vi "CustomSpectrum.vi"(0 "LightField Automation":refnum<class "LightField Automation.lvclass">, 1 "Photodiode handle out":refnum<visa-resource-name> caption="instrument handle out", 3 "Stop Spectrum Custom":refnum<vi>, 4 "Photodiode error out":errorcluster caption="error out" {"code" format="%.0x"}, 5 "LightField Automation error":errorcluster, 6 "CCD 1D Spectrum Main":refnum<vi>, 7 "Center Wavelength (nm)":refnum<vi>, 8 "Scan Spectrum Progess Bar":refnum<vi>, 10 "Excitation Power (uW)":refnum<vi>, 12 "Scan Spectrum Cust Exp Params 2":T1) -> (11 "WLs":dbl[](array[numeric]), 13 "PL":dbl[](array[numeric]), 14 "LFA Out":refnum<class "LightField Automation.lvclass">, 15 "PD Out":refnum<visa-resource-name>, 17 "movemonotime":u32, 18 "PD Error Our":errorcluster, 19 "LFA Error Out":errorcluster)   [LabVIEW 2019]
uses:
  C:/Users/manip/Documents/Controle_Manip_2020/Thorlabs.MotionControl.KCube.SolenoidCLI.dll
  Thorlabs.MotionControl.KCube.SolenoidCLI.dll
  Light Field/lightfield-automation-labview/LightField Automation.lvclass
  <vilib>/Analysis/baseanly.llb/Mean (DBL).vi
  <vilib>/Analysis/NI_AALBase.lvlib
panel:
  in  "Scan Spectrum Progess Bar":u8(slide) scale=0.0..100.0
  in  "Stop Spectrum Custom 2":bool
  in  "Stop Spectrum Custom":bool
  out "Array 2":i32[](array[numeric])
  out "Array":dbl[](array[numeric])
  out "Acq Time (ms)":dbl
  out "NumPoints":dbl
  out "KCube Shutter On?":bool
  out "Spectrum Custom Mode":u16
  out "Spectrum End Wavelength (nm)":dbl
  out "Spectrum Step Wavelength (nm)":dbl
  out "Spectrum Start Wavelength (nm)":dbl
  in  "Scan Spectrum Cust Exp Params":T2
  in  "Center Wavelength (nm)":dbl=490.12 caption="Center WL :"
  out "Excitation Power (uW)":dbl=0.2 caption="P    =" format="%#_3p"
  out "CCD 1D Spectrum Main":cluster{dbl[], dbl[]}(graph)
  out "Shutter Ctrls":u16(ring)
  out "KCube Shutter Device Reference":refnum<k24>
types:
  T1 = cluster{"Acq Time (ms)":dbl, "Spectrum Start Wavelength (nm)":dbl, "Spectrum Step Wavelength (nm)":dbl, "Spectrum End Wavelength (nm)":dbl, "Spectrum Custom Mode":u16, "KCube Shutter On?":bool}
  T2 = cluster{"Spectrum Start Wavelength (nm)":dbl, "Spectrum Step Wavelength (nm)":dbl, "Spectrum End Wavelength (nm)":dbl, "Spectrum Custom Mode":u16, "KCube Shutter On?":bool}
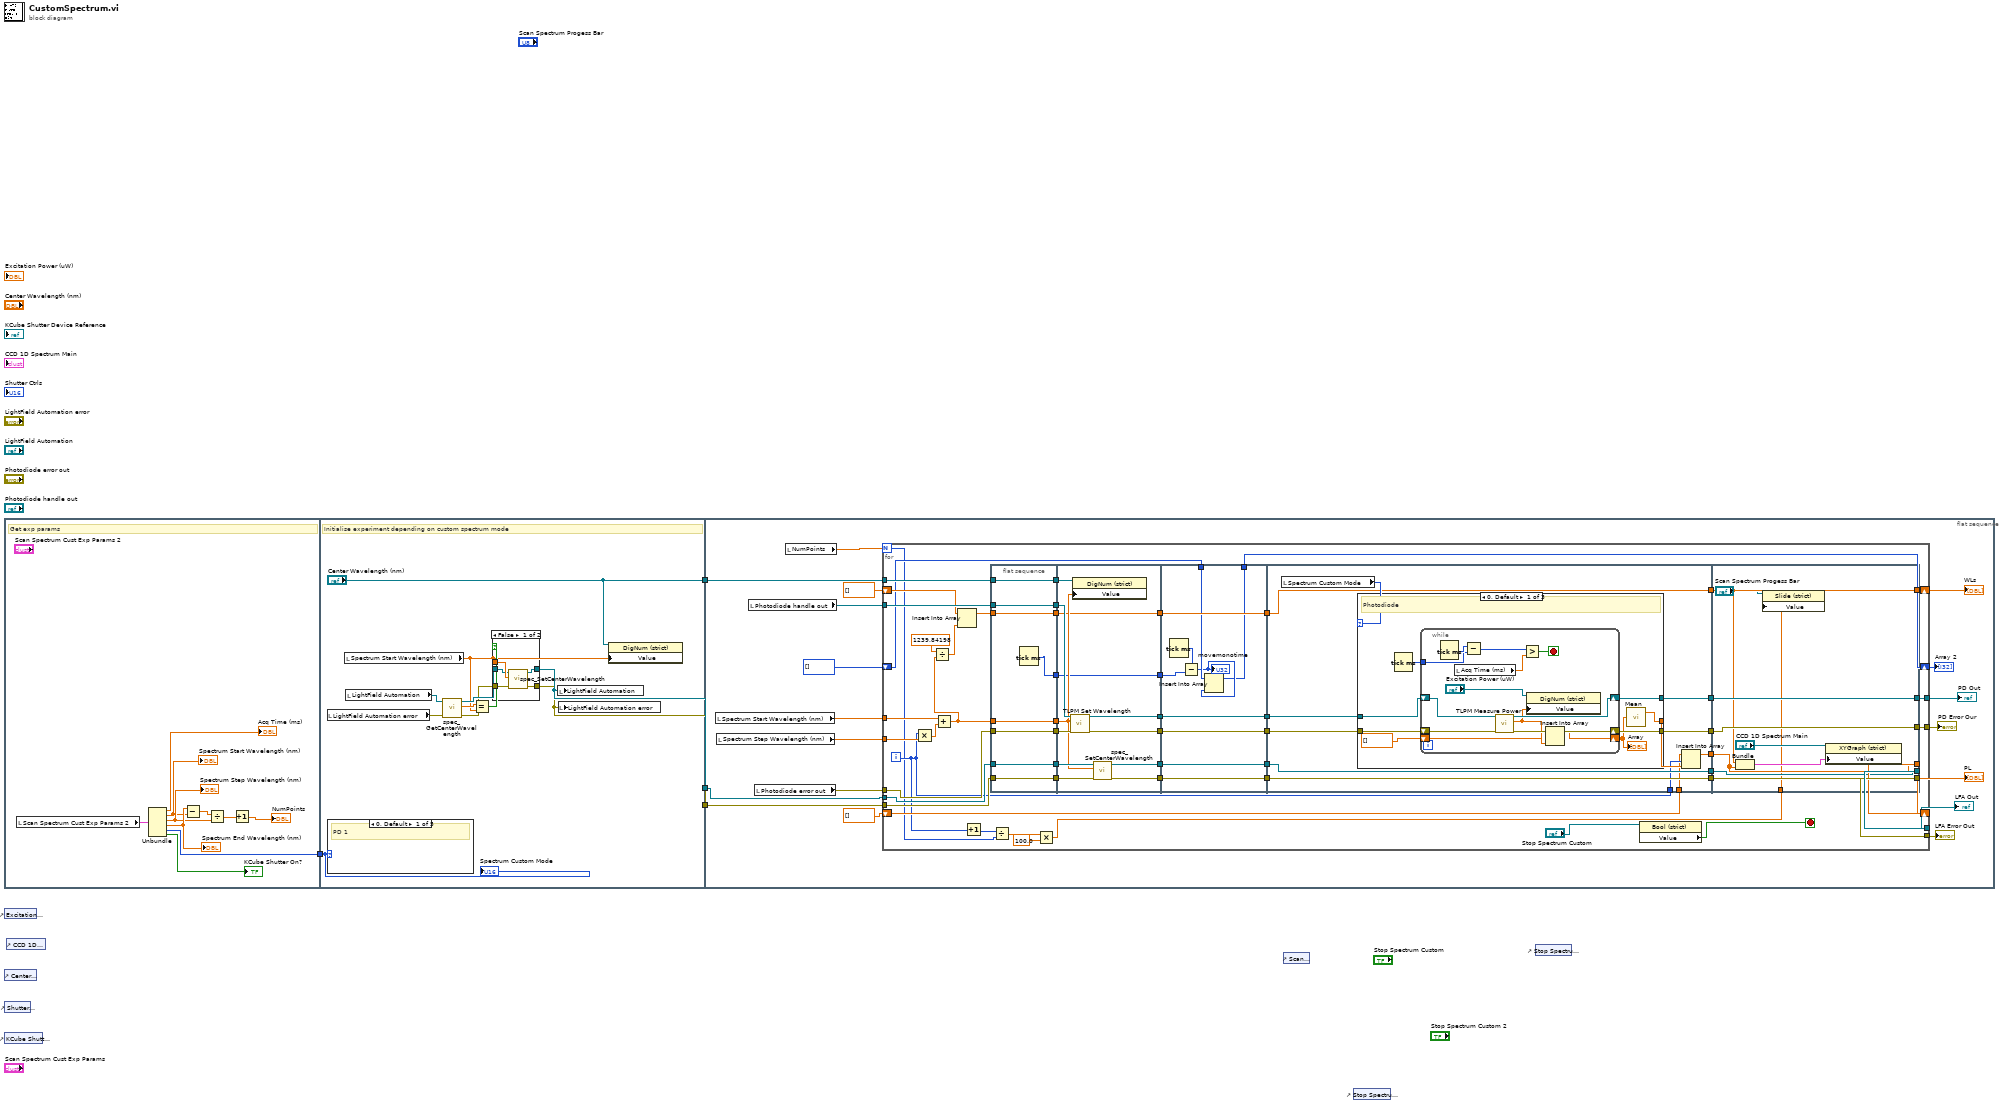
[diagram p0: block diagram]
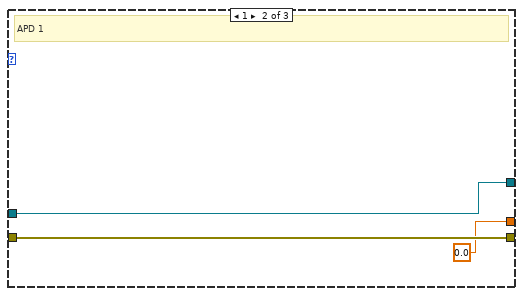
[diagram p7: hidden frame]
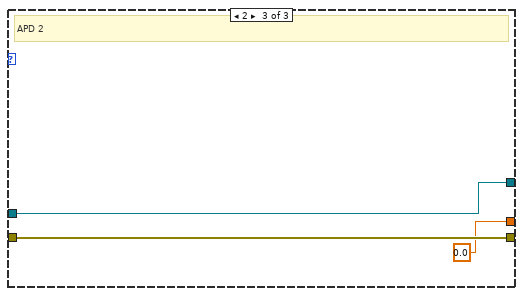
[diagram p8: hidden frame]
diagram:
  n1 = flat-sequence {
    tunnel: [w9] -> w4
    tunnel: w4 -> [w25]
    tunnel: [w17] -> w3
    tunnel: [w16] -> w2
    tunnel: ["Center Wavelength (nm)"] -> w1
    tunnel: w3 -> [w44]
    tunnel: w2 -> [w42]
    tunnel: w1 -> [w39]
    frame #0 {
      # "Get exp params"
      n2 = local read "Scan Spectrum Cust Exp Params 2"() -> (w14:T1)
      n3 = Unbundle(w14) -> ("Acq Time (ms)"=→"Acq Time (ms)":dbl, "Spectrum Start Wavelength (nm)"=w6:dbl, "Spectrum Step Wavelength (nm)"=w7:dbl, "Spectrum End Wavelength (nm)"=w8:dbl, "Spectrum Custom Mode"=w9:u16, "KCube Shutter On?"=→"KCube Shutter On?":bool)
      "Spectrum Start Wavelength (nm)" <- w6
      "Spectrum Step Wavelength (nm)" <- w7
      "Spectrum End Wavelength (nm)" <- w8
      n4 = Subtract(x=w8, y=w6) -> (x-y=w13:dbl)
      n5 = Divide(x=w13, y=w7) -> (x/y=w12:dbl)
      n6 = Increment(x=w12) -> (x+1=→"NumPoints":dbl)
    }
    frame #1 {
      # "Initialise experiment depending on custom spectrum mode"
      n7 = local read "LightField Automation error"() -> (w23:errorcluster)
      n8 = case shown="0, Default" w25 {
        frame 0, Default {
          # "PD 1"
        }
        frame 1 {
          # "APD 1"
        }
        frame 2 {
          # "APD 2"
        }
        frame 3 {
          # "APD 1+2"
        }
        frame 4 {
          # "PD 2"
        }
      }
      n9 = local read "Spectrum Start Wavelength (nm)"() -> (w18:dbl)
      n10 = local read "LightField Automation"() -> (w24:refnum<class "LightField Automation.lvclass">)
      n11 = call "spec_GetCenterWavelength.vi"("error in (no error)"=w23, "LightField Automation in"=w24) -> ("error out"=w19:errorcluster, "Center Wavelength"=w22:dbl, "LightField Automation out"=w20:refnum<class "LightField Automation.lvclass">)  [unwired: 7 in]
      n12 = Equal?(x=w22, y=w18) -> (x = y?=w21:bool)
      n13 = case shown="False" w21 {
        tunnel: w20 -> [w28 w32]
        tunnel: w19 -> [w29 w31]
        tunnel: [w27 w32] -> w17
        tunnel: [w26 w31] -> w16
        tunnel: w18 -> [w30 _]
        frame False {
          n14 = call "spec_SetCenterWavelength.vi"("error in (no error)"=w29, "Center Wavelength"=w30, "LightField Automation in"=w28) -> ("error out"=w26:errorcluster, "LightField Automation out"=w27:refnum<class "LightField Automation.lvclass">)  [unwired: 7 in]
        }
        frame True {
        }
      }
      n15 = local write "LightField Automation"(w17) -> ()
      n16 = local write "LightField Automation error"(w16) -> ()
      n17 = property class="DigNum (strict)"(reference="Center Wavelength (nm)", "Value"=w18) -> ()  [unwired: 1 in, 2 out]
      "Spectrum Custom Mode" <- w25
    }
    frame #2 {
      n18 = local read "Spectrum Start Wavelength (nm)"() -> (w49:dbl)
      n19 = local read "Spectrum Step Wavelength (nm)"() -> (w50:dbl)
      n20 = local read "Photodiode handle out"() -> (w45:refnum<visa-resource-name>)
      n21 = local read "Photodiode error out"() -> (w46:errorcluster)
      n22 = local read "NumPoints"() -> (w40:dbl)
      n23 = for {
        N: w40 -> [w57]
        tunnel: w50 -> [w104]
        tunnel: w49 -> [w103]
        tunnel: [w94] -> w48
        tunnel: [w93] -> w47
        tunnel: w46 -> [w92]
        tunnel: w45 -> [w91]
        tunnel: w44 -> [w90]
        tunnel: [w89] -> w43
        tunnel: w42 -> [w88]
        tunnel: [w87] -> w41
        tunnel: w39 -> [w86]
        shift-right: [w73] -> w36
        shift-left: dbl[] [] -> [w77]
        shift-right: [w74] -> w35
        shift-left: dbl[] [] -> [w75]
        shift-right: [w62] -> w33
        shift-left: i32[] [] -> [w63]
        i -> [w59]
        stop <- w60 stop-if-true
        n24 = Multiply(x=w59, y=w104) -> (x*y=w105:dbl)
        n25 = Add(x=w103, y=w105) -> (x+y=w52:dbl)
        n26 = Divide(x=1239.84198, y=w52) -> (x/y=w51:dbl)
        n27 = Insert Into Array(array=w77, new element=w51) -> (w76:dbl[])  [unwired: 1 in]
        n28 = Increment(x=w59) -> (x+1=w58:i32)
        n29 = flat-sequence {
          tunnel: w76 -> [w107]
          tunnel: w86 -> [w108]
          tunnel: w91 -> [w109]
          tunnel: w92 -> [w110]
          tunnel: w88 -> [w111]
          tunnel: w90 -> [w112]
          tunnel: w52 -> [w113]
          tunnel: [w113] -> w72
          tunnel: [w112] -> w71
          tunnel: [w111] -> w70
          tunnel: [w110] -> w69
          tunnel: [w109] -> w68
          tunnel: [w108] -> w67
          tunnel: [w107] -> w66
          tunnel: [w106] -> w65
          tunnel: [w123] -> w101
          tunnel: [w122] -> w100
          tunnel: [w121] -> w97
          tunnel: [w120] -> w95
          tunnel: [w115] -> w80
          tunnel: w72 -> [w117]
          tunnel: w71 -> [w125]
          tunnel: w70 -> [w124]
          tunnel: w69 -> [w119]
          tunnel: w68 -> [w118]
          tunnel: w67 -> [w116]
          tunnel: w66 -> [w115]
          tunnel: w65 -> [w114]
          tunnel: [w114] -> w64
          tunnel: [w135] -> w102
          tunnel: w101 -> [w135]
          tunnel: w100 -> [w134]
          tunnel: [w134] -> w99
          tunnel: [w133] -> w98
          tunnel: w97 -> [w133]
          tunnel: [w132] -> w96
          tunnel: w95 -> [w132]
          tunnel: w80 -> [w131]
          tunnel: [w131] -> w79
          tunnel: w64 -> [w129]
          tunnel: w63 -> [w128]
          tunnel: [w126] -> w62
          tunnel: w102 -> [w146]
          tunnel: w99 -> [w145]
          tunnel: w98 -> [w142]
          tunnel: w96 -> [w141]
          tunnel: w75 -> [w136]
          tunnel: w59 -> [w139]
          tunnel: [w144] -> w85
          tunnel: [w143] -> w84
          tunnel: [w142] -> w83
          tunnel: [w141] -> w82
          tunnel: [w138] -> w81
          tunnel: w79 -> [w137]
          tunnel: [w137] -> w78
          tunnel: [w181] -> w87
          tunnel: [w182] -> w89
          tunnel: [w183] -> w94
          tunnel: [w184] -> w93
          tunnel: w85 -> [w184]
          tunnel: w84 -> [w183]
          tunnel: w83 -> [w182]
          tunnel: w82 -> [w181]
          tunnel: w81 -> [w177]
          tunnel: w78 -> [w178]
          tunnel: [w178] -> w73
          tunnel: [w177] -> w74
          tunnel: w54 -> [w175]
          frame #0 {
            n30 = Tick Count (ms)() -> (millisecond timer value=w106:u32)
          }
          frame #1 {
            n31 = call <instrlib>:"TLPM Set Wavelength.vi"("error in (no error)"=w119, "Wavelength (0.0)"=w117, "instrument handle"=w118) -> ("error out"=w122:errorcluster, "instrument handle out"=w123:refnum<visa-resource-name>)  [unwired: 7 in]
            n32 = property class="DigNum (strict)"(reference=w116, "Value"=w117) -> ()  [unwired: 1 in, 2 out]
            n33 = call "spec_SetCenterWavelength.vi"("error in (no error)"=w124, "Center Wavelength"=w117, "LightField Automation in"=w125) -> ("error out"=w120:errorcluster, "LightField Automation out"=w121:refnum<class "LightField Automation.lvclass">)  [unwired: 7 in]
          }
          frame #2 {
            n34 = Tick Count (ms)() -> (millisecond timer value=w130:u32)
            n35 = Subtract(x=w130, y=w129) -> (x-y=w127:u32)
            "movemonotime" <- w127
            n36 = Insert Into Array(array=w128, new element=w127) -> (w126:i32[])  [unwired: 1 in]
          }
          frame #3 {
            n37 = local read "Spectrum Custom Mode"() -> (w147:u16)
            n38 = case shown="0, Default" w147 {
              tunnel: w146 -> [w155 w171 w174]
              tunnel: w145 -> [w154 w170 w173]
              tunnel: [w153 w170 w173] -> w144
              tunnel: [w152 w171 w174] -> w143
              tunnel: [w148 0.0 ("Power") 0.0 ("Power")] -> w140
              frame 0, Default {
                # "Photodiode"
                n39 = Tick Count (ms)() -> (millisecond timer value=w151:u32)
                n40 = while {
                  shift-right: [w165] -> w152
                  shift-left: w155 -> [w168]
                  shift-right: [w166] -> w153
                  shift-left: w154 -> [w167]
                  tunnel: w151 -> [w162]
                  shift-right: [w156] -> w149
                  shift-left: dbl[] [] -> [w157]
                  stop <- w159 stop-if-true
                  n41 = Tick Count (ms)() -> (millisecond timer value=w163:u32)
                  n42 = local read "Acq Time (ms)"() -> (w160:dbl)
                  n43 = Subtract(x=w163, y=w162) -> (x-y=w161:u32)
                  n44 = call <instrlib>:"TLPM Measure Power.vi"("error in (no error)"=w167, "instrument handle"=w168) -> ("error out"=w166:errorcluster, "Power"=w158:dbl, "instrument handle out"=w165:refnum<visa-resource-name>)  [unwired: 7 in]
                  n45 = Greater?(x=w161, y=w160) -> (0:w159:bool)
                  n46 = property class="DigNum (strict)"(reference="Excitation Power (uW)", "Value"=w158) -> ()  [unwired: 1 in, 2 out]
                  n47 = Insert Into Array(array=w157, new element=w158) -> (w156:dbl[])  [unwired: 1 in]
                }
                "Array" <- w149
                n48 = call-poly <vilib>:"Mean.vi"("X"=w149) -> ("mean"=w148:dbl)  [unwired: 1 out]
              }
              frame 1 {
                # "APD 1"
              }
              frame 2 {
                # "APD 2"
              }
            }
            n49 = Insert Into Array(array=w136, index=w139, new element=w140) -> (w138:dbl[])
          }
          frame #4 {
            n50 = Bundle(w178, w177) -> (w180:cluster{dbl[], dbl[]})  [unwired: 1 in]
            n51 = property class="Slide (strict)"(reference="Scan Spectrum Progess Bar", "Value"=w175) -> ()  [unwired: 1 in, 2 out]
            n52 = property class="XYGraph (strict)"(reference="CCD 1D Spectrum Main", "Value"=w180) -> ()  [unwired: 1 in, 2 out]
          }
        }
        n53 = Divide(x=w58, y=w57) -> (x/y=w56:dbl)
        n54 = Multiply(x=w56, y=100.0) -> (x*y=w54:dbl)
        n55 = property class="Bool (strict)"(reference="Stop Spectrum Custom") -> ("Value"=w60:bool)  [unwired: 1 in, 2 out]
      }
      "PD Out" <- w48
      "PD Error Our" <- w47
      "LFA Out" <- w43
      "LFA Error Out" <- w41
      "WLs" <- w36
      "PL" <- w35
      "Array 2" <- w33
    }
  }
  n56 = control-ref of="Excitation Power (uW)"() -> ()  [unwired: 1 out]
  n57 = control-ref of="Center Wavelength (nm)"() -> ()  [unwired: 1 out]
  n58 = control-ref of="Shutter Ctrls"() -> ()  [unwired: 1 out]
  n59 = control-ref of="KCube Shutter Device Reference"() -> ()  [unwired: 1 out]
  n60 = control-ref of="CCD 1D Spectrum Main"() -> ()  [unwired: 1 out]
  n61 = control-ref of="Scan Spectrum Progess Bar"() -> ()  [unwired: 1 out]
  n62 = control-ref of="Stop Spectrum Custom"() -> ()  [unwired: 1 out]
  n63 = control-ref of="Stop Spectrum Custom 2"() -> ()  [unwired: 1 out]
